vi "IMAQ-SaveVideo.vi"(1 "Exposure Time (ms)":u32, 2 "Image":T1, 3 "Grabar":refnum<vi>, 4 "Compression Filter":string) -> (0 "Selected Path for AVI":path)   [LabVIEW 2010]
uses:
  <vilib>/vision/Image Controls.llb/IMAQ Image.ctl
  <vilib>/vision/Avi1.llb/AviRefnum.ctl
  <vilib>/Utility/error.llb/DialogType.ctl
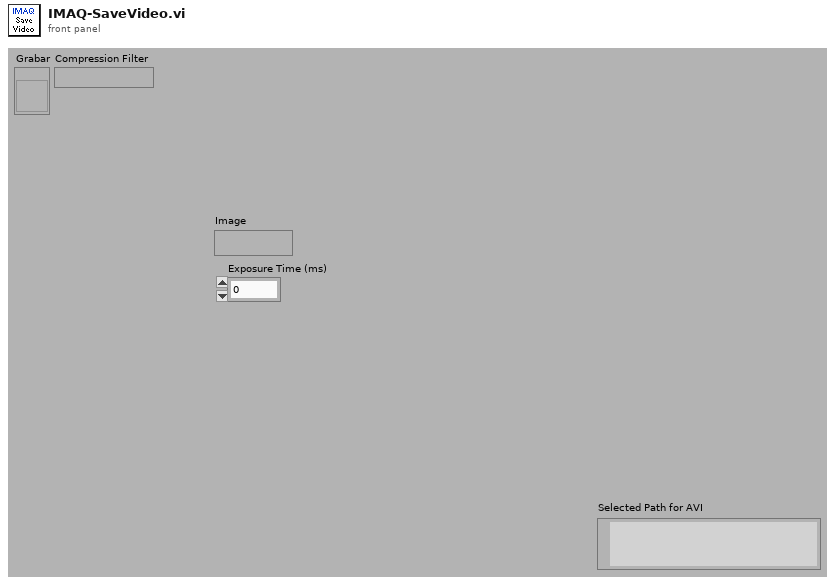
[diagram p1: front panel]
types:
  T1 = typedef "IMAQ Image.ctl" = refnum<image>
  T2 = typedef "AviRefnum.ctl" = refnum<k1>
  T3 = enum32{"existing file", "new file", "new or existing file", "existing dir", "new dir", "new or existing dir", "existing file (use LLBs)", "new file (use LLBs)", "new or existing file (use LLBs)", "new or existing file or directory (use LLBs)"}
  T4 = typedef "DialogType.ctl" = u16
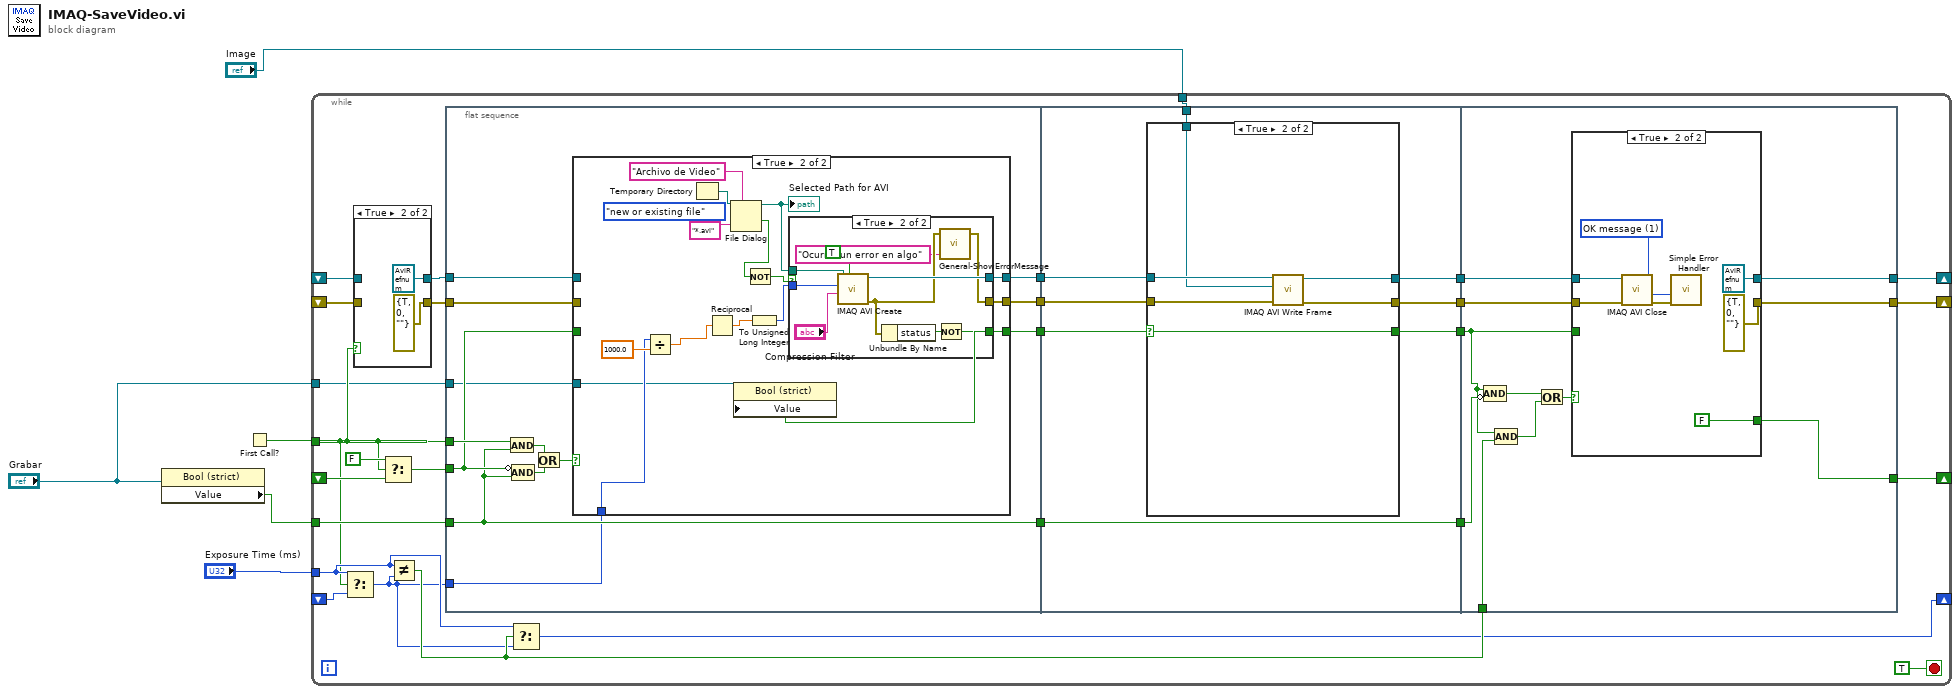
[diagram p0: block diagram]
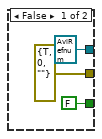
[diagram p4: hidden frame]
diagram:
  n1 = property class="Bool (strict)"(reference="Grabar") -> ("Value"=w2:bool)  [unwired: 1 in, 2 out]
  n2 = First Call?() -> (First Call?: T/F=w5:bool)
  n3 = while {
    tunnel: w5 -> [w7]
    tunnel: w2 -> [w32]
    shift-right: [w17] -> _
    shift-left: _ -> [w30]
    tunnel: "Image" -> [w26]
    shift-right: [w22] -> _
    shift-left: _ -> [w10]
    shift-right: [w21] -> _
    shift-left: _ -> [w8]
    tunnel: "Exposure Time (ms)" -> [w14]
    shift-right: [w12] -> _
    shift-left: _ -> [w16]
    tunnel: "Grabar" -> [w6]
    stop <- TRUE stop-if-true
    n4 = Select(t=w14, s=w7, f=w16) -> (s? t:f=w13:u32)
    n5 = case shown="True" w7 {
      tunnel: [w35 T2 refnum ("Avi Refnum (duplicate)")] -> w11
      tunnel: w10 -> [w35 _]
      tunnel: [w34 errorcluster {"status"=TRUE, "code"=0, "source"=""} ("error out")] -> w9
      tunnel: w8 -> [w34 _]
      frame False {
      }
      frame True {
      }
    }
    n6 = Select(t=FALSE, s=w7, f=w30) -> (s? t:f=w29:bool)
    n7 = Not Equal?(x=w14, y=w13) -> (x != y?=w15:bool)
    n8 = flat-sequence {
      tunnel: w7 -> [w47]
      tunnel: w32 -> [w40]
      tunnel: w29 -> [w43]
      tunnel: [w46] -> w28
      tunnel: [w45] -> w27
      tunnel: [w44] -> w25
      tunnel: w11 -> [w42]
      tunnel: w9 -> [w41]
      tunnel: [w40] -> w20
      tunnel: w13 -> [w39]
      tunnel: w6 -> [w38]
      tunnel: w28 -> [w89]
      tunnel: w27 -> [w88]
      tunnel: w26 -> [w87]
      tunnel: w25 -> [w86]
      tunnel: [w85] -> w24
      tunnel: [w84] -> w23
      tunnel: w20 -> [w83]
      tunnel: [w83] -> w19
      tunnel: [w82] -> w18
      tunnel: w24 -> [w109]
      tunnel: w23 -> [w108]
      tunnel: [w107] -> w22
      tunnel: [w106] -> w21
      tunnel: w19 -> [w105]
      tunnel: w18 -> [w100]
      tunnel: [w104] -> w17
      tunnel: w15 -> [w101]
      frame #0 {
        n9 = And(x=w47, y=w40) -> (x .and. y?=w49:bool)
        n10 = Compound Arithmetic op=AND(invert w43, w40) -> (w48:bool)
        n11 = Or(x=w49, y=w48) -> (x .or. y?=w50:bool)
        n12 = case shown="True" w50 {
          tunnel: [w51 w56] -> w46
          tunnel: [w52 w60] -> w45
          tunnel: [w53 w57] -> w44
          tunnel: w43 -> [w53 _]
          tunnel: w42 -> [w52 _]
          tunnel: w41 -> [w51 _]
          tunnel: w39 -> [_ w59]
          tunnel: w38 -> [_ w58]
          frame False {
          }
          frame True {
            (unwired) T3."new or existing file" ("select mode (2)")
            n13 = Divide(x=w59, y=1000.0) -> (x/y=w63:dbl)
            n14 = Temporary Directory() -> (w66:path)
            n15 = Reciprocal(x=w63) -> (1/x=w62:dbl)
            n16 = File Dialog(6:"*.avi" ("pattern"), 7:"Archivo de Video" ("prompt"), 11:w66) -> (1:w54:bool, 3:w65:path)  [unwired: 1 in, 5 out]
            "Selected Path for AVI" <- w65
            n17 = Not(x=w54) -> (.not. x?=w55:bool)
            n18 = To Unsigned Long Integer(number=w62) -> (unsigned 32bit integer=w61:u32)
            n19 = case shown="True" w55 {
              tunnel: w65 -> [_ w81]
              tunnel: w61 -> [_ w79]
              tunnel: [T2 refnum ("Avi Refnum") w77] -> w60
              tunnel: [FALSE w76] -> w57
              tunnel: [errorcluster {"status"=TRUE, "code"=0, "source"=""} ("Error OUT") w74] -> w56
              frame False {
              }
              frame True {
                n20 = call "IMAQ AVI Create"("Has Data"=TRUE, "Compression Filter"="Compression Filter", "Frames Per Second"=w79, "AVI Path"=w81) -> ("error out"=w75:errorcluster, "Avi Refnum"=w77:T2)  [unwired: 6 in]
                n21 = Unbundle By Name(w75) -> ("status"=w78:bool)
                n22 = Not(x=w78) -> (.not. x?=w76:bool)
                n23 = call "General-ShowErrorMessage.vi"("message"="Ocurrio un error en algo", "Error IN"=w75) -> ("Error OUT"=w74:errorcluster)  [unwired: 3 in]
              }
            }
            n24 = property class="Bool (strict)"(reference=w58, "Value"=w57) -> ()  [unwired: 1 in, 2 out]
          }
        }
      }
      frame #1 {
        n25 = case shown="True" w86 {
          selector: w86 -> [w90 w93]
          tunnel: w89 -> [w91 w98]
          tunnel: w88 -> [w92 w97]
          tunnel: w87 -> [_ w96]
          tunnel: [w91 w95] -> w85
          tunnel: [w92 w94] -> w84
          tunnel: [w90 w93] -> w82
          frame False {
          }
          frame True {
            n26 = call "IMAQ AVI Write Frame"("error in (no error)"=w98, "Image"=w96, "Avi Refnum"=w97) -> ("error out"=w95:errorcluster, "Avi Refnum (duplicate)"=w94:T2)  [unwired: 1 in, 6 out]
          }
        }
      }
      frame #2 {
        n27 = Compound Arithmetic op=AND(w100, invert w105) -> (w103:bool)
        n28 = Compound Arithmetic op=AND(w100, w101) -> (w99:bool)
        n29 = Or(x=w103, y=w99) -> (x .or. y?=w102:bool)
        n30 = case shown="True" w102 {
          tunnel: w109 -> [w111 w117]
          tunnel: w108 -> [w112 w118]
          tunnel: [w112 T2 refnum ("Avi Refnum (duplicate)")] -> w107
          tunnel: [w111 errorcluster {"status"=TRUE, "code"=0, "source"=""} ("error out")] -> w106
          tunnel: [w110 FALSE] -> w104
          tunnel: w100 -> [w110 _]
          frame False {
          }
          frame True {
            w113 = T4 1 items=["no dialog", "OK message", "continue or stop message", "OK message + warnings", "continue/stop + warnings"] ("type of dialog (OK msg:1)")
            n31 = call "IMAQ AVI Close"("error in (no error)"=w117, "Avi Refnum"=w118) -> ("error out"=w119:errorcluster)  [unwired: 9 out]
            n32 = call <vilib>:"Simple Error Handler.vi"("type of dialog (OK msg:1)"=w113, "error in (no error)"=w119) -> ()  [unwired: 8 out]
          }
        }
      }
    }
    n33 = Select(t=w14, s=w15, f=w13) -> (s? t:f=w12:u32)
  }
